vi "Test Micro Master.vi"() -> ()   [LabVIEW 2023]
uses:
  Modbus TCP Micro Master/Modbus TCP Micro Master.lvclass
panel:
  out "Regular Data":T1
  out "Read Values":u16[](array[numeric])
  out "x-y":u32
  in  "Stop":bool
  out "Discrete Inputs":bool[](array[boolean])
  out "Array 2":u16[](array[numeric])
  out "Array":u16[](array[numeric])
  out "Coil States":bool[](array[boolean])
  out "error out":errorcluster
  in  "error in (no error)":errorcluster
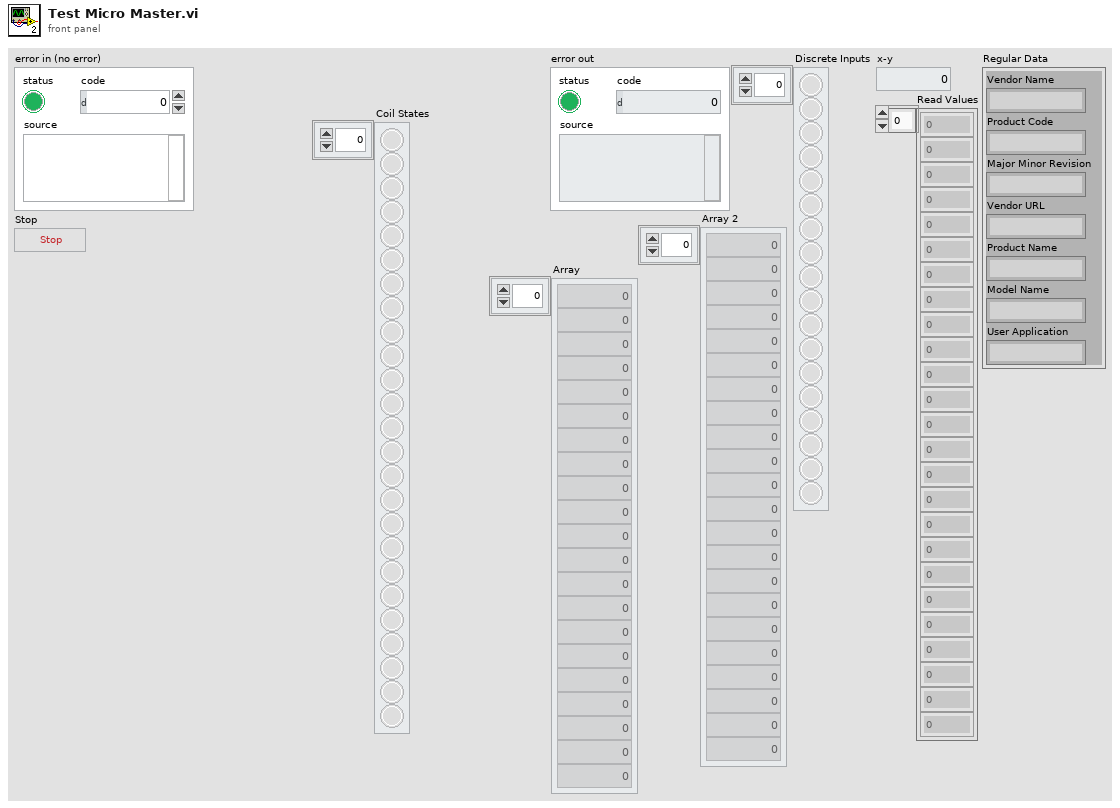
[diagram p1: front panel]
types:
  T1 = cluster{"Vendor Name":string, "Product Code":string, "Major Minor Revision":string, "Vendor URL":string, "Product Name":string, "Model Name":string, "User Application":string}
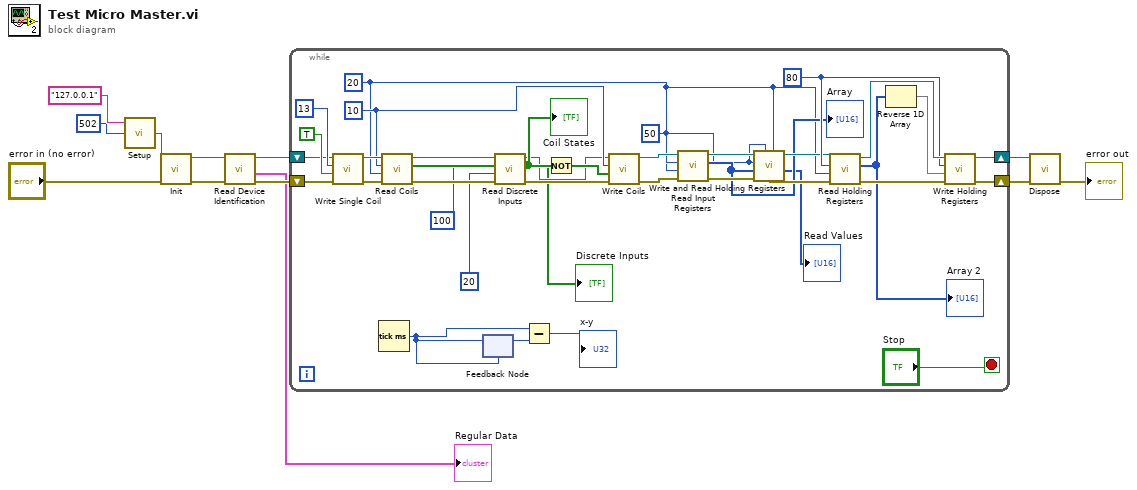
[diagram p0: block diagram]
diagram:
  n1 = call "Setup.vi"("Remote Port (502)"=u16 502 ("remote port or service name"), "slave host"="127.0.0.1" ("address")) -> ("Modbus TCP Micro Master out"=w5:refnum<class "Modbus TCP Micro Master.lvclass">)  [unwired: 2 in]
  n2 = call "Init.vi"("error in (no error)"="error in (no error)", "Modbus TCP Micro Master in"=w5) -> ("error out"=w10:errorcluster, "Modbus TCP Micro Master out"=w3:refnum<class "Modbus TCP Micro Master.lvclass">)  [unwired: 8 in]
  n3 = call "Read Device Identification.vi"("error in (no error)"=w10, "Modbus TCP Micro Master in"=w3) -> ("error out"=w4:errorcluster, "Regular Data"=→"Regular Data":T1, "Modbus TCP Micro Master out"=w2:refnum<class "Modbus TCP Micro Master.lvclass">)  [unwired: 6 in, 1 out]
  n4 = while {
    shift-right: [w41] -> w9
    shift-left: w4 -> [w48]
    shift-right: [w39] -> w8
    shift-left: w2 -> [w31]
    stop <- "Stop" stop-if-true
    w38 = u16 80 ("Start Address")
    w14 = u16 50 ("Start Address")
    w13 = u16 20 ("Number of Registers")
    w34 = u16 10 ("Start Address")
    n5 = call "Write Single Coil.vi"("error in (no error)"=w48, "Value"=TRUE, "Address"=u16 13 ("Start Address"), "Modbus TCP Micro Master in"=w31) -> ("error out"=w49:errorcluster, "Modbus TCP Micro Master out"=w42:refnum<class "Modbus TCP Micro Master.lvclass">)  [unwired: 6 in]
    n6 = Tick Count (ms)() -> (millisecond timer value=w22:u32)
    n7 = call "Read Coils.vi"("error in (no error)"=w49, "Number of Registers"=w13, "Start Address"=w34, "Modbus TCP Micro Master in"=w42) -> ("error out"=w45:errorcluster, "Coil States"=w33:bool[], "Modbus TCP Micro Master out"=w29:refnum<class "Modbus TCP Micro Master.lvclass">)  [unwired: 5 in]
    "Coil States" <- w33
    n8 = feedback-in #1(w22) -> ()
    n9 = feedback #1(w22) -> (w23:u32)
    n10 = call "Read Discrete Inputs.vi"("error in (no error)"=w45, "Number of Registers"=u16 20, "Start Address"=u16 100, "Modbus TCP Micro Master in"=w29) -> ("error out"=w30:errorcluster, "Coil States"=→"Discrete Inputs":bool[], "Modbus TCP Micro Master out"=w28:refnum<class "Modbus TCP Micro Master.lvclass">)  [unwired: 5 in]
    n11 = Subtract(x=w22, y=w23) -> (x-y=→"x-y":u32)
    n12 = Not(x=w33) -> (.not. x?=w32:bool[])
    n13 = call "Write Coils.vi"("error in (no error)"=w30, "Values"=w32, "Start Address"=w34, "Modbus TCP Micro Master in"=w28) -> ("error out"=w35:errorcluster, "Modbus TCP Micro Master out"=w20:refnum<class "Modbus TCP Micro Master.lvclass">)  [unwired: 6 in]
    n14 = call "Read Input Registers.vi"("error in (no error)"=w35, "Number of Registers"=w13, "Start Address"=w14, "Modbus TCP Micro Master in"=w20) -> ("error out"=w44:errorcluster, "Input Registers"=w16:u16[], "Modbus TCP Micro Master out"=w18:refnum<class "Modbus TCP Micro Master.lvclass">)  [unwired: 5 in]
    "Array" <- w16
    n15 = call "Write and Read Holding Registers.vi"("Read Count"=w13, "Read Start Address"=w14, "error in (no error)"=w44, "Write Values"=w16, "Start Address"=w14, "Modbus TCP Micro Master in"=w18) -> ("error out"=w19:errorcluster, "Read Values"=→"Read Values":u16[], "Modbus TCP Micro Master out"=w17:refnum<class "Modbus TCP Micro Master.lvclass">)  [unwired: 3 in]
    n16 = call "Read Holding Registers.vi"("error in (no error)"=w19, "Number of Registers"=w13, "Start Address"=w38, "Modbus TCP Micro Master in"=w17) -> ("error out"=w43:errorcluster, "Holding Registers"=w37:u16[], "Modbus TCP Micro Master out"=w40:refnum<class "Modbus TCP Micro Master.lvclass">)  [unwired: 5 in]
    "Array 2" <- w37
    n17 = Reverse 1D Array(array=w37) -> (reversed array=w36:u16[])
    n18 = call "Write Holding Registers.vi"("error in (no error)"=w43, "Values"=w36, "Start Address"=w38, "Modbus TCP Micro Master in"=w40) -> ("error out"=w41:errorcluster, "Modbus TCP Micro Master out"=w39:refnum<class "Modbus TCP Micro Master.lvclass">)  [unwired: 6 in]
  }
  n19 = call "Dispose.vi"("error in (no error)"=w9, "Modbus TCP Micro Master in"=w8) -> ("error out"=→"error out":errorcluster)  [unwired: 9 in]
